vi "Get Result Status.vi"(8 "error in (no error)":errorcluster, 11 "Execution in":refnum<class "Execution.lvclass">) -> (0 "error out":errorcluster, 2 "Result Status":string, 3 "Execution out":refnum<class "Execution.lvclass">)   [LabVIEW 2020, in "TSnax.lvlib" / "Execution.lvclass"]
uses:
  Execution.lvclass
  Execution.lvclass/Execution.ctl
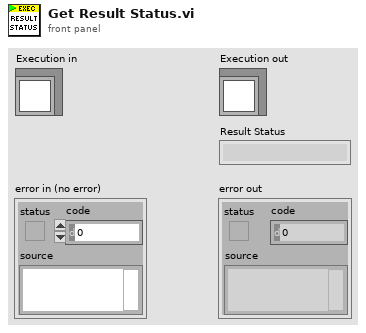
[diagram p1: front panel]
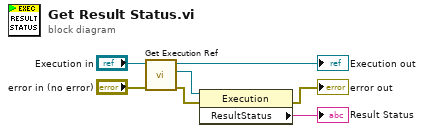
[diagram p0: block diagram]
diagram:
  n1 = call "Get Execution Ref.vi"("error in (no error)"="error in (no error)", "Execution in"="Execution in") -> ("error out"=w3:errorcluster, "Execution Ref"=w5:refnum<k7>, "Execution out"=→"Execution out":refnum<class "Execution.lvclass">)  [unwired: 7 in]
  n2 = property class="Execution"(reference=w5, error in=w3) -> (error out=→"error out":errorcluster, "ResultStatus"=→"Result Status":string)  [unwired: 1 out]
